vi "Get All Elements.vi"(8 "error in":errorcluster, 10 "Channel Node":refnum<k20>, 11 "Channel Ref in":refnum<data-value>) -> (0 "error out":errorcluster, 3 "Channel Ref out":refnum<data-value>)   [LabVIEW 2024, in "Config File Parser.lvlib" / "Channel.lvclass"]
uses:
  Channel.lvclass
  C:/dev/CD/CD 2.0/Config-File-Parser/Item/Item.lvclass
  Channel.lvclass/Channel.ctl
  <vilib>/xml/Close Reference(Node).vi
  Config File Parser.lvlib
  <resource>/objmgr/DOMUserDefRef.rc
  <vilib>/xml/NI_XML.lvlib
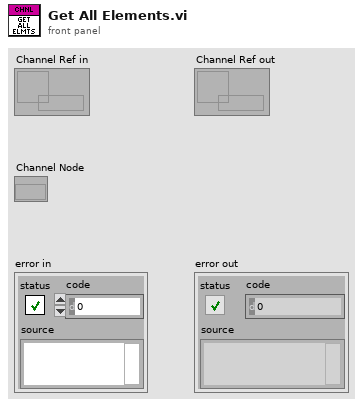
[diagram p1: front panel]
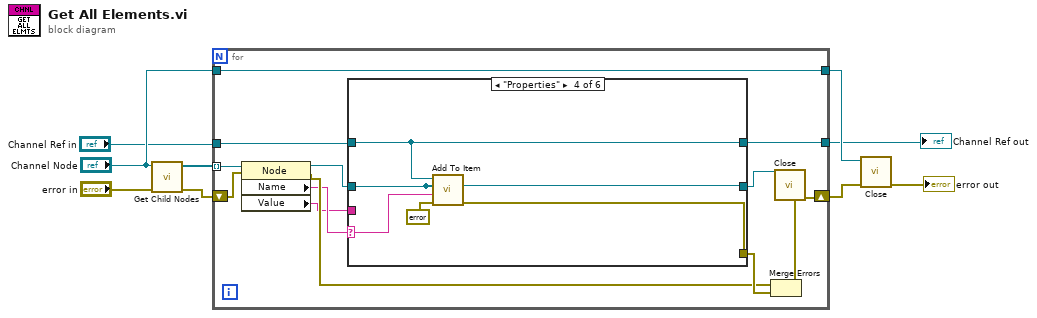
[diagram p0: block diagram]
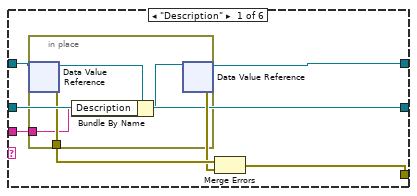
[diagram p2: hidden frame]
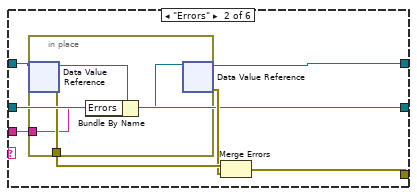
[diagram p3: hidden frame]
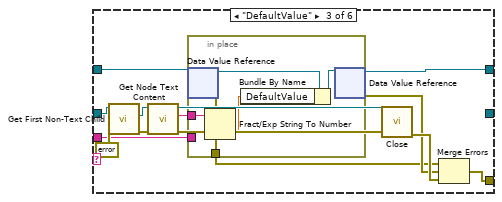
[diagram p4: hidden frame]
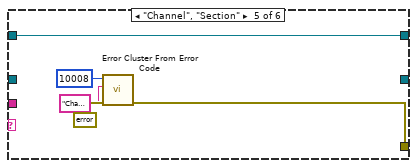
[diagram p5: hidden frame]
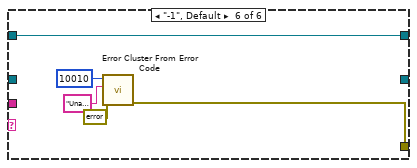
[diagram p6: hidden frame]
diagram:
  n1 = call "Get Child Nodes.vi"("error in"="error in", "Node"="Channel Node") -> ("error out"=w8:errorcluster, "Child Nodes"=w5:refnum<k20>[])  [unwired: 8 in]
  n2 = for {
    tunnel: w5 -> [w17] mode=indexing
    shift-right: [w21] -> w7
    shift-left: w8 -> [w22]
    tunnel: [w13] -> w4
    tunnel: "Channel Node" -> [w13]
    tunnel: "Channel Ref in" -> [w11]
    tunnel: [w10] -> w1
    n3 = property class="Node"(reference=w17, error in=w22) -> (reference out=w15:refnum<k20>, error out=w19:errorcluster, "Name"=w16:string, "Value"=w14:string)
    n4 = case shown="\"Properties\"" w16 {
      selector: w16 -> [_ _ _ w66 _ _]
      tunnel: w15 -> [w24 w35 w48 w65 _ _]
      tunnel: w14 -> [w25 w36 w50 _ _ _]
      tunnel: [w24 w35 _ w65 _ _] -> w12
      tunnel: w11 -> [w26 w37 w51 w64 w69 w74]
      tunnel: [w29 w40 w53 w68 w72 w77] -> w20
      tunnel: [w23 w34 w49 w64 w69 w74] -> w10
      frame "Description" {
        n5 = in-place {
          in-place-border: w25 -> [w31]
          in-place-border: [w33] -> w28
          n6 = in-place-dvr #1(w26) -> (w32:refnum<class "Channel.lvclass">, w33:errorcluster)
          n7 = Bundle By Name(cluster=w32, "Description"=w31) -> (w30:refnum<class "Channel.lvclass">)
          n8 = in-place-dvr #1(w30) -> (w23:refnum<data-value>, w27:errorcluster)
        }
        n9 = Merge Errors(w28, w27) -> (w29:errorcluster)
      }
      frame "Errors" {
        n10 = in-place {
          in-place-border: w36 -> [w42]
          in-place-border: [w44] -> w39
          n11 = in-place-dvr #2(w37) -> (w43:refnum<class "Channel.lvclass">, w44:errorcluster)
          n12 = Bundle By Name(cluster=w43, "Errors"=w42) -> (w41:refnum<class "Channel.lvclass">)
          n13 = in-place-dvr #2(w41) -> (w34:refnum<data-value>, w38:errorcluster)
        }
        n14 = Merge Errors(w39, w38) -> (w40:errorcluster)
      }
      frame "DefaultValue" {
        n15 = call <vilib>:"Get First Non-Text Child.vi"("error in (no error)"=errorcluster {"status"=FALSE, "code"=0, "source"=""}, "node in"=w48) -> ("error out"=w57:errorcluster, "child node"=w47:refnum<k20>)  [unwired: 6 in, 2 out]
        n16 = call <vilib>:"Get Node Text Content.vi"("error in (no error)"=w57, "node in"=w47) -> ("error out"=w56:errorcluster, "node text"=w46:string, "node out"=w45:refnum<k20>)  [unwired: 7 in]
        n17 = in-place {
          in-place-border: w50 -> [_]
          in-place-border: [w63] -> w52
          in-place-border: w46 -> [w60]
          n18 = in-place-dvr #3(w51) -> (w62:refnum<class "Channel.lvclass">, w63:errorcluster)
          n19 = Fract/Exp String To Number(string=w60) -> (number=w59:dbl)  [unwired: 3 in, 1 out]
          n20 = Bundle By Name(cluster=w62, "DefaultValue"=w59) -> (w61:refnum<class "Channel.lvclass">)
          n21 = in-place-dvr #3(w61) -> (w49:refnum<data-value>, w54:errorcluster)
        }
        n22 = call-poly <vilib>:"Close.vi"("error in (no error)"=w56, "node"=w45) -> ("error out"=w55:errorcluster)  [unwired: 7 in]
        n23 = Merge Errors(w52, w54, w55) -> (w53:errorcluster)
      }
      frame "Properties" {
        n24 = call "Add To Item.vi"("error in"=errorcluster {"status"=FALSE, "code"=0, "source"=""}, "Item Name"=w66, "Item node"=w65, "Parent Item Ref in"=w64) -> ("error out"=w68:errorcluster)  [unwired: 6 in, 1 out]
      }
      frame "Channel", "Section" {
        n25 = call <vilib>:"Error Cluster From Error Code.vi"("error in (no error)"=errorcluster {"status"=FALSE, "code"=0, "source"=""}, "error message (\"\")"="Channel should not contains channels or sections in it", "error code (0)"=10008) -> ("error out"=w72:errorcluster)  [unwired: 6 in]
      }
      frame "-1", Default {
        n26 = call <vilib>:"Error Cluster From Error Code.vi"("error in (no error)"=errorcluster {"status"=FALSE, "code"=0, "source"=""}, "error message (\"\")"="Unauthorized elements are found. The channel should not contain any unauthorized elements", "error code (0)"=10010) -> ("error out"=w77:errorcluster)  [unwired: 6 in]
      }
    }
    n27 = Merge Errors(w19, w20) -> (w18:errorcluster)
    n28 = call-poly <vilib>:"Close.vi"("error in (no error)"=w18, "node"=w12) -> ("error out"=w21:errorcluster)  [unwired: 7 in]
  }
  "Channel Ref out" <- w1
  n29 = call-poly <vilib>:"Close.vi"("error in (no error)"=w7, "node"=w4) -> ("error out"=→"error out":errorcluster)  [unwired: 7 in]
